vi "Destroy.vi"(8 "Error In":errorcluster, 11 "reference in":refnum<class "Fetch Waveforms CFG.lvclass">) -> (0 "Error Out":errorcluster, 3 "reference out":refnum<class "Fetch Waveforms CFG.lvclass">)   [LabVIEW 2023, in "Scope Simulated.lvlib" / "Fetch Waveforms CFG.lvclass"]
uses:
  Fetch Waveforms CFG.lvclass
  Configuration Base/Configuration Base.lvclass
  Fetch Waveforms CFG.lvclass/Fetch Waveforms CFG.ctl
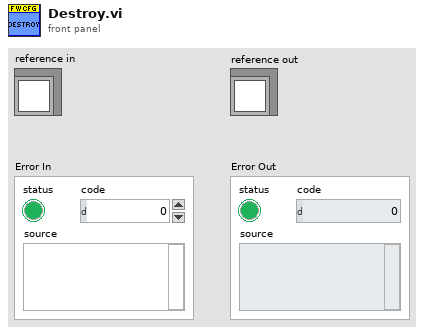
[diagram p1: front panel]
types:
  T1 = typedef "G4BaseTemplate_Simple_4x4x4.lvclass/ObjectAttributes.ctl" = cluster{"Attribute1":dbl}
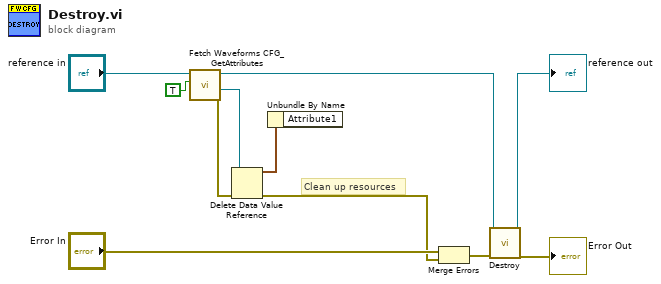
[diagram p0: block diagram]
diagram:
  # "Clean up resources"
  n1 = call "Fetch Waveforms CFG_GetAttributes.vi"("OnlyGetDvrReference(False)"=TRUE, "reference in"="reference in") -> ("Error Out"=w9:errorcluster, "DataRef"=w7:refnum<data-value>, "reference out"=w8:refnum<class "Fetch Waveforms CFG.lvclass">)  [unwired: 6 in, 1 out]
  n2 = Delete Data Value Reference(data value reference=w7, error in=w9) -> (data value=w1:T1, error out=w5:errorcluster)
  n3 = Unbundle By Name(w1) -> ()  [unwired: 1 out]
  n4 = Merge Errors("Error In", w5) -> (w11:errorcluster)
  n5 = call-parent "Destroy.vi"("Error In"=w11, "reference in"=w8) -> ("Error Out"=→"Error Out":errorcluster, "reference out"=→"reference out":refnum<class "Fetch Waveforms CFG.lvclass">)  [unwired: 8 in]
